vi "FeedbackDecode_SetMvntBuilder.vi"(2 "MvntBuilderIn":T1={"MvntType"={"Thumb"=enum."True", "Index"=enum."False", "Middle"=enum."False", "Ring"=enum."False", "Little"=enum."False", "ThumbInt"=enum."False", "IndexInt"=enum."False", "RingInt"=enum."False", "LittleInt"=enum."False", "WristPitch"=enum."False", "WristYaw"=enum."False", "WristRoll"=enum."False"}, "MvntParams"={"Amp"=1.0, "Delay"=0.0, "Rise"=1.0, "Hold"=1.0}, "MvntList"=[{"MvntMat"=[[1.0, 0.0, 1.0, 1.0], [0.0, 0.0, 0.0, 0.0], [0.0, 0.0, 0.0, 0.0], [0.0, 0.0, 0.0, 0.0], [0.0, 0.0, 0.0, 0.0], [0.0, 0.0, 0.0, 0.0], [0.0, 0.0, 0.0, 0.0], [0.0, 0.0, 0.0, 0.0], [0.0, 0.0, 0.0, 0.0], [0.0, 0.0, 0.0, 0.0], [0.0, 0.0, 0.0, 0.0], [0.0, 0.0, 0.0, 0.0]], "MvntName"="ThumbFlex", "Tracking"=enum."False", "Radius"=0.15}, {"MvntMat"=[[0.0, 0.0, 0.0, 0.0], [1.0, 0.0, 2.0, 2.0], [0.0, 0.0, 0.0, 0.0], [0.0, 0.0, 0.0, 0.0], [0.0, 0.0, 0.0, 0.0], [0.0, 0.0, 0.0, 0.0], [0.0, 0.0, 0.0, 0.0], [0.0, 0.0, 0.0, 0.0], [0.0, 0.0, 0.0, 0.0], [0.0, 0.0, 0.0, 0.0], [0.0, 0.0, 0.0, 0.0], [0.0, 0.0, 0.0, 0.0]], "MvntName"="IndexFlex", "Tracking"=enum."True", "Radius"=0.15}, {"MvntMat"=[[0.0, 0.0, 0.0, 0.0], [0.0, 0.0, 0.0, 0.0], [1.0, 0.0, 1.0, 1.0], [0.0, 0.0, 0.0, 0.0], [0.0, 0.0, 0.0, 0.0], [0.0, 0.0, 0.0, 0.0], [0.0, 0.0, 0.0, 0.0], [0.0, 0.0, 0.0, 0.0], [0.0, 0.0, 0.0, 0.0], [0.0, 0.0, 0.0, 0.0], [0.0, 0.0, 0.0, 0.0], [0.0, 0.0, 0.0, 0.0]], "MvntName"="MiddleFlex", "Tracking"=enum."False", "Radius"=0.15}, {"MvntMat"=[[0.0, 0.0, 0.0, 0.0], [0.0, 0.0, 0.0, 0.0], [0.0, 0.0, 0.0, 0.0], [1.0, 0.0, 1.0, 1.0], [0.0, 0.0, 0.0, 0.0], [0.0, 0.0, 0.0, 0.0], [0.0, 0.0, 0.0, 0.0], [0.0, 0.0, 0.0, 0.0], [0.0, 0.0, 0.0, 0.0], [0.0, 0.0, 0.0, 0.0], [0.0, 0.0, 0.0, 0.0], [0.0, 0.0, 0.0, 0.0]], "MvntName"="RingFlex", "Tracking"=enum."False", "Radius"=0.15}, {"MvntMat"=[[0.0, 0.0, 0.0, 0.0], [0.0, 0.0, 0.0, 0.0], [0.0, 0.0, 0.0, 0.0], [0.0, 0.0, 0.0, 0.0], [1.0, 0.0, 1.0, 1.0], [0.0, 0.0, 0.0, 0.0], [0.0, 0.0, 0.0, 0.0], [0.0, 0.0, 0.0, 0.0], [0.0, 0.0, 0.0, 0.0], [0.0, 0.0, 0.0, 0.0], [0.0, 0.0, 0.0, 0.0], [0.0, 0.0, 0.0, 0.0]], "MvntName"="LittleFlex", "Tracking"=enum."False", "Radius"=0.15}, {"MvntMat"=[[0.0, 0.0, 0.0, 0.0], [0.0, 0.0, 0.0, 0.0], [0.0, 0.0, 0.0, 0.0], [0.0, 0.0, 0.0, 0.0], [0.0, 0.0, 0.0, 0.0], [1.0, 0.0, 1.0, 1.0], [0.0, 0.0, 0.0, 0.0], [0.0, 0.0, 0.0, 0.0], [0.0, 0.0, 0.0, 0.0], [0.0, 0.0, 0.0, 0.0], [0.0, 0.0, 0.0, 0.0], [0.0, 0.0, 0.0, 0.0]], "MvntName"="ThumbInt", "Tracking"=enum."False", "Radius"=0.15}, {"MvntMat"=[[0.0, 0.0, 0.0, 0.0], [0.0, 0.0, 0.0, 0.0], [0.0, 0.0, 0.0, 0.0], [0.0, 0.0, 0.0, 0.0], [0.0, 0.0, 0.0, 0.0], [0.0, 0.0, 0.0, 0.0], [1.0, 0.0, 1.0, 1.0], [0.0, 0.0, 0.0, 0.0], [0.0, 0.0, 0.0, 0.0], [0.0, 0.0, 0.0, 0.0], [0.0, 0.0, 0.0, 0.0], [0.0, 0.0, 0.0, 0.0]], "MvntName"="IndexInt", "Tracking"=enum."False", "Radius"=0.15}, {"MvntMat"=[[0.0, 0.0, 0.0, 0.0], [0.0, 0.0, 0.0, 0.0], [0.0, 0.0, 0.0, 0.0], [0.0, 0.0, 0.0, 0.0], [0.0, 0.0, 0.0, 0.0], [0.0, 0.0, 0.0, 0.0], [0.0, 0.0, 0.0, 0.0], [1.0, 0.0, 1.0, 1.0], [0.0, 0.0, 0.0, 0.0], [0.0, 0.0, 0.0, 0.0], [0.0, 0.0, 0.0, 0.0], [0.0, 0.0, 0.0, 0.0]], "MvntName"="RingInt", "Tracking"=enum."False", "Radius"=0.15}, {"MvntMat"=[[0.0, 0.0, 0.0, 0.0], [0.0, 0.0, 0.0, 0.0], [0.0, 0.0, 0.0, 0.0], [0.0, 0.0, 0.0, 0.0], [0.0, 0.0, 0.0, 0.0], [0.0, 0.0, 0.0, 0.0], [0.0, 0.0, 0.0, 0.0], [0.0, 0.0, 0.0, 0.0], [1.0, 0.0, 1.0, 1.0], [0.0, 0.0, 0.0, 0.0], [0.0, 0.0, 0.0, 0.0], [0.0, 0.0, 0.0, 0.0]], "MvntName"="LittleInt", "Tracking"=enum."False", "Radius"=0.15}, {"MvntMat"=[[0.0, 0.0, 0.0, 0.0], [0.0, 0.0, 0.0, 0.0], [0.0, 0.0, 0.0, 0.0], [0.0, 0.0, 0.0, 0.0], [0.0, 0.0, 0.0, 0.0], [0.0, 0.0, 0.0, 0.0], [0.0, 0.0, 0.0, 0.0], [0.0, 0.0, 0.0, 0.0], [0.0, 0.0, 0.0, 0.0], [1.0, 0.0, 1.0, 1.0], [0.0, 0.0, 0.0, 0.0], [0.0, 0.0, 0.0, 0.0]], "MvntName"="WristPitch", "Tracking"=enum."False", "Radius"=0.15}, {"MvntMat"=[[0.0, 0.0, 0.0, 0.0], [0.0, 0.0, 0.0, 0.0], [0.0, 0.0, 0.0, 0.0], [0.0, 0.0, 0.0, 0.0], [0.0, 0.0, 0.0, 0.0], [0.0, 0.0, 0.0, 0.0], [0.0, 0.0, 0.0, 0.0], [0.0, 0.0, 0.0, 0.0], [0.0, 0.0, 0.0, 0.0], [0.0, 0.0, 0.0, 0.0], [1.0, 0.0, 1.0, 1.0], [0.0, 0.0, 0.0, 0.0]], "MvntName"="WristYaw", "Tracking"=enum."False", "Radius"=0.15}, {"MvntMat"=[[0.0, 0.0, 0.0, 0.0], [0.0, 0.0, 0.0, 0.0], [0.0, 0.0, 0.0, 0.0], [0.0, 0.0, 0.0, 0.0], [0.0, 0.0, 0.0, 0.0], [0.0, 0.0, 0.0, 0.0], [0.0, 0.0, 0.0, 0.0], [0.0, 0.0, 0.0, 0.0], [0.0, 0.0, 0.0, 0.0], [0.0, 0.0, 0.0, 0.0], [0.0, 0.0, 0.0, 0.0], [1.0, 0.0, 1.0, 1.0]], "MvntName"="WristRoll", "Tracking"=enum."False", "Radius"=0.15}], "Set"=FALSE, "Clear"=FALSE, "Load"=FALSE, "Mode"=enum."Selected", "NTrials"=0.0, "TargParams"={"Gain"=1.0, "Radius"=0.15, "Acc"=0.8}, "Save"=FALSE, "PercTrials"=1.0} caption="Movement Builder" {"PercTrials" format="%#_2g"; "NTrials" min=1.0 max=100.0 step=1.0; "MvntList"."Radius" min=0.0 max=1.0 step=0.01; "TargParams"."Acc" min=0.0 max=1.0 step=0.01; "TargParams"."Radius" min=0.0 max=1.0 step=0.01; "TargParams"."Gain" min=-1.0 max=1.0 step=0.01; "MvntParams"."Hold" min=0.0 step=0.1; "MvntParams"."Rise" min=0.0 step=0.1; "MvntParams"."Delay" min=0.0 step=0.1; "MvntParams"."Amp" min=-1.0 max=1.0 step=0.1}, 3 "MvntIdx":i32) -> (0 "MvntBuilderOut":T1={"MvntType"={"Thumb"=enum."True", "Index"=enum."False", "Middle"=enum."False", "Ring"=enum."False", "Little"=enum."False", "ThumbInt"=enum."False", "IndexInt"=enum."False", "RingInt"=enum."False", "LittleInt"=enum."False", "WristPitch"=enum."False", "WristYaw"=enum."False", "WristRoll"=enum."False"}, "MvntParams"={"Amp"=1.0, "Delay"=0.0, "Rise"=1.0, "Hold"=1.0}, "MvntList"=[{"MvntMat"=[[1.0, 0.0, 1.0, 1.0], [0.0, 0.0, 0.0, 0.0], [0.0, 0.0, 0.0, 0.0], [0.0, 0.0, 0.0, 0.0], [0.0, 0.0, 0.0, 0.0], [0.0, 0.0, 0.0, 0.0], [0.0, 0.0, 0.0, 0.0], [0.0, 0.0, 0.0, 0.0], [0.0, 0.0, 0.0, 0.0], [0.0, 0.0, 0.0, 0.0], [0.0, 0.0, 0.0, 0.0], [0.0, 0.0, 0.0, 0.0]], "MvntName"="ThumbFlex", "Tracking"=enum."False", "Radius"=0.15}, {"MvntMat"=[[0.0, 0.0, 0.0, 0.0], [1.0, 0.0, 2.0, 2.0], [0.0, 0.0, 0.0, 0.0], [0.0, 0.0, 0.0, 0.0], [0.0, 0.0, 0.0, 0.0], [0.0, 0.0, 0.0, 0.0], [0.0, 0.0, 0.0, 0.0], [0.0, 0.0, 0.0, 0.0], [0.0, 0.0, 0.0, 0.0], [0.0, 0.0, 0.0, 0.0], [0.0, 0.0, 0.0, 0.0], [0.0, 0.0, 0.0, 0.0]], "MvntName"="IndexFlex", "Tracking"=enum."True", "Radius"=0.15}, {"MvntMat"=[[0.0, 0.0, 0.0, 0.0], [0.0, 0.0, 0.0, 0.0], [1.0, 0.0, 1.0, 1.0], [0.0, 0.0, 0.0, 0.0], [0.0, 0.0, 0.0, 0.0], [0.0, 0.0, 0.0, 0.0], [0.0, 0.0, 0.0, 0.0], [0.0, 0.0, 0.0, 0.0], [0.0, 0.0, 0.0, 0.0], [0.0, 0.0, 0.0, 0.0], [0.0, 0.0, 0.0, 0.0], [0.0, 0.0, 0.0, 0.0]], "MvntName"="MiddleFlex", "Tracking"=enum."False", "Radius"=0.15}, {"MvntMat"=[[0.0, 0.0, 0.0, 0.0], [0.0, 0.0, 0.0, 0.0], [0.0, 0.0, 0.0, 0.0], [1.0, 0.0, 1.0, 1.0], [0.0, 0.0, 0.0, 0.0], [0.0, 0.0, 0.0, 0.0], [0.0, 0.0, 0.0, 0.0], [0.0, 0.0, 0.0, 0.0], [0.0, 0.0, 0.0, 0.0], [0.0, 0.0, 0.0, 0.0], [0.0, 0.0, 0.0, 0.0], [0.0, 0.0, 0.0, 0.0]], "MvntName"="RingFlex", "Tracking"=enum."False", "Radius"=0.15}, {"MvntMat"=[[0.0, 0.0, 0.0, 0.0], [0.0, 0.0, 0.0, 0.0], [0.0, 0.0, 0.0, 0.0], [0.0, 0.0, 0.0, 0.0], [1.0, 0.0, 1.0, 1.0], [0.0, 0.0, 0.0, 0.0], [0.0, 0.0, 0.0, 0.0], [0.0, 0.0, 0.0, 0.0], [0.0, 0.0, 0.0, 0.0], [0.0, 0.0, 0.0, 0.0], [0.0, 0.0, 0.0, 0.0], [0.0, 0.0, 0.0, 0.0]], "MvntName"="LittleFlex", "Tracking"=enum."False", "Radius"=0.15}, {"MvntMat"=[[0.0, 0.0, 0.0, 0.0], [0.0, 0.0, 0.0, 0.0], [0.0, 0.0, 0.0, 0.0], [0.0, 0.0, 0.0, 0.0], [0.0, 0.0, 0.0, 0.0], [1.0, 0.0, 1.0, 1.0], [0.0, 0.0, 0.0, 0.0], [0.0, 0.0, 0.0, 0.0], [0.0, 0.0, 0.0, 0.0], [0.0, 0.0, 0.0, 0.0], [0.0, 0.0, 0.0, 0.0], [0.0, 0.0, 0.0, 0.0]], "MvntName"="ThumbInt", "Tracking"=enum."False", "Radius"=0.15}, {"MvntMat"=[[0.0, 0.0, 0.0, 0.0], [0.0, 0.0, 0.0, 0.0], [0.0, 0.0, 0.0, 0.0], [0.0, 0.0, 0.0, 0.0], [0.0, 0.0, 0.0, 0.0], [0.0, 0.0, 0.0, 0.0], [1.0, 0.0, 1.0, 1.0], [0.0, 0.0, 0.0, 0.0], [0.0, 0.0, 0.0, 0.0], [0.0, 0.0, 0.0, 0.0], [0.0, 0.0, 0.0, 0.0], [0.0, 0.0, 0.0, 0.0]], "MvntName"="IndexInt", "Tracking"=enum."False", "Radius"=0.15}, {"MvntMat"=[[0.0, 0.0, 0.0, 0.0], [0.0, 0.0, 0.0, 0.0], [0.0, 0.0, 0.0, 0.0], [0.0, 0.0, 0.0, 0.0], [0.0, 0.0, 0.0, 0.0], [0.0, 0.0, 0.0, 0.0], [0.0, 0.0, 0.0, 0.0], [1.0, 0.0, 1.0, 1.0], [0.0, 0.0, 0.0, 0.0], [0.0, 0.0, 0.0, 0.0], [0.0, 0.0, 0.0, 0.0], [0.0, 0.0, 0.0, 0.0]], "MvntName"="RingInt", "Tracking"=enum."False", "Radius"=0.15}, {"MvntMat"=[[0.0, 0.0, 0.0, 0.0], [0.0, 0.0, 0.0, 0.0], [0.0, 0.0, 0.0, 0.0], [0.0, 0.0, 0.0, 0.0], [0.0, 0.0, 0.0, 0.0], [0.0, 0.0, 0.0, 0.0], [0.0, 0.0, 0.0, 0.0], [0.0, 0.0, 0.0, 0.0], [1.0, 0.0, 1.0, 1.0], [0.0, 0.0, 0.0, 0.0], [0.0, 0.0, 0.0, 0.0], [0.0, 0.0, 0.0, 0.0]], "MvntName"="LittleInt", "Tracking"=enum."False", "Radius"=0.15}, {"MvntMat"=[[0.0, 0.0, 0.0, 0.0], [0.0, 0.0, 0.0, 0.0], [0.0, 0.0, 0.0, 0.0], [0.0, 0.0, 0.0, 0.0], [0.0, 0.0, 0.0, 0.0], [0.0, 0.0, 0.0, 0.0], [0.0, 0.0, 0.0, 0.0], [0.0, 0.0, 0.0, 0.0], [0.0, 0.0, 0.0, 0.0], [1.0, 0.0, 1.0, 1.0], [0.0, 0.0, 0.0, 0.0], [0.0, 0.0, 0.0, 0.0]], "MvntName"="WristPitch", "Tracking"=enum."False", "Radius"=0.15}, {"MvntMat"=[[0.0, 0.0, 0.0, 0.0], [0.0, 0.0, 0.0, 0.0], [0.0, 0.0, 0.0, 0.0], [0.0, 0.0, 0.0, 0.0], [0.0, 0.0, 0.0, 0.0], [0.0, 0.0, 0.0, 0.0], [0.0, 0.0, 0.0, 0.0], [0.0, 0.0, 0.0, 0.0], [0.0, 0.0, 0.0, 0.0], [0.0, 0.0, 0.0, 0.0], [1.0, 0.0, 1.0, 1.0], [0.0, 0.0, 0.0, 0.0]], "MvntName"="WristYaw", "Tracking"=enum."False", "Radius"=0.15}, {"MvntMat"=[[0.0, 0.0, 0.0, 0.0], [0.0, 0.0, 0.0, 0.0], [0.0, 0.0, 0.0, 0.0], [0.0, 0.0, 0.0, 0.0], [0.0, 0.0, 0.0, 0.0], [0.0, 0.0, 0.0, 0.0], [0.0, 0.0, 0.0, 0.0], [0.0, 0.0, 0.0, 0.0], [0.0, 0.0, 0.0, 0.0], [0.0, 0.0, 0.0, 0.0], [0.0, 0.0, 0.0, 0.0], [1.0, 0.0, 1.0, 1.0]], "MvntName"="WristRoll", "Tracking"=enum."False", "Radius"=0.15}], "Set"=FALSE, "Clear"=FALSE, "Load"=FALSE, "Mode"=enum."Selected", "NTrials"=0.0, "TargParams"={"Gain"=1.0, "Radius"=0.15, "Acc"=0.8}, "Save"=FALSE, "PercTrials"=1.0} caption="Movement Builder" {"PercTrials" format="%#_2g"; "NTrials" min=1.0 max=100.0 step=1.0; "MvntList"."Radius" min=0.0 max=1.0 step=0.01; "TargParams"."Acc" min=0.0 max=1.0 step=0.01; "TargParams"."Radius" min=0.0 max=1.0 step=0.01; "TargParams"."Gain" min=-1.0 max=1.0 step=0.01; "MvntParams"."Hold" min=0.0 step=0.1; "MvntParams"."Rise" min=0.0 step=0.1; "MvntParams"."Delay" min=0.0 step=0.1; "MvntParams"."Amp" min=-1.0 max=1.0 step=0.1})   [LabVIEW 2020]
uses:
  FeedbackDecode_MvntClust.ctl
panel:
  # "Thumb"
  # "Index"
  # "Middle"
  # "Ring"
  # "Little"
  # "ThumbInt"
  # "IndexInt"
  # "RingInt"
  # "LittleInt"
  # "WristPitch"
  # "WristYaw"
  # "WristRoll"
  # "Amp"
  # "Del"
  # "Rise"
  # "Hold"
  # "Thumb"
  # "Index"
  # "Middle"
  # "Ring"
  # "Little"
  # "ThumbInt"
  # "IndexInt"
  # "RingInt"
  # "LittleInt"
  # "WristPitch"
  # "WristYaw"
  # "WristRoll"
  # "Amp"
  # "Del"
  # "Rise"
  # "Hold"
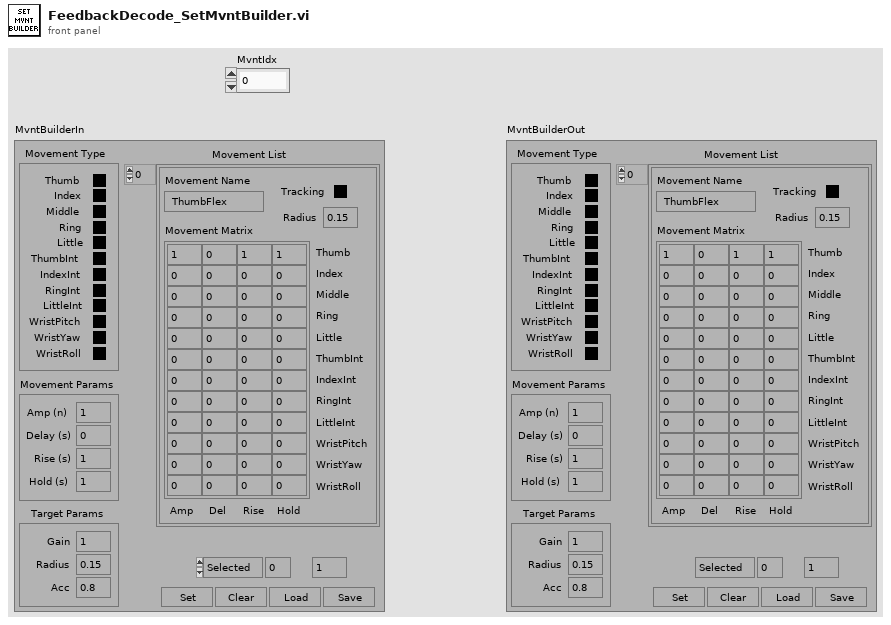
[diagram p1: front panel]
types:
  T1 = typedef "FeedbackDecode_MvntClust.ctl" = cluster{"MvntType":cluster{"Thumb":enum8{"False", "True", "Mixed"}, "Index":enum8{"False", "True", "Mixed"}, "Middle":enum8{"False", "True", "Mixed"}, "Ring":enum8{"False", "True", "Mixed"}, "Little":enum8{"False", "True", "Mixed"}, "ThumbInt":enum8{"False", "True", "Mixed"}, "IndexInt":enum8{"False", "True", "Mixed"}, "RingInt":enum8{"False", "True", "Mixed"}, "LittleInt":enum8{"False", "True", "Mixed"}, "WristPitch":enum8{"False", "True", "Mixed"}, "WristYaw":enum8{"False", "True", "Mixed"}, "WristRoll":enum8{"False", "True", "Mixed"}}, "MvntParams":cluster{"Amp":dbl, "Delay":dbl, "Rise":dbl, "Hold":dbl}, "MvntList":cluster{"MvntMat":dbl[][], "MvntName":string, "Tracking":enum8{"False", "True", "Mixed"}, "Radius":dbl}[], "Set":bool, "Clear":bool, "Load":bool, "Mode":enum16{"Selected", "Block", "Random"}, "NTrials":dbl, "TargParams":cluster{"Gain":dbl, "Radius":dbl, "Acc":dbl}, "Save":bool, "PercTrials":dbl}
  T2 = cluster{"Thumb":enum8{"False", "True", "Mixed"}, "Index":enum8{"False", "True", "Mixed"}, "Middle":enum8{"False", "True", "Mixed"}, "Ring":enum8{"False", "True", "Mixed"}, "Little":enum8{"False", "True", "Mixed"}, "ThumbInt":enum8{"False", "True", "Mixed"}, "IndexInt":enum8{"False", "True", "Mixed"}, "RingInt":enum8{"False", "True", "Mixed"}, "LittleInt":enum8{"False", "True", "Mixed"}, "WristPitch":enum8{"False", "True", "Mixed"}, "WristYaw":enum8{"False", "True", "Mixed"}, "WristRoll":enum8{"False", "True", "Mixed"}}
  T3 = cluster{"Amp":dbl, "Delay":dbl, "Rise":dbl, "Hold":dbl}
  T4 = cluster{"MvntMat":dbl[][], "MvntName":string, "Tracking":enum8{"False", "True", "Mixed"}, "Radius":dbl}[]
  T5 = cluster{"MvntMat":dbl[][], "MvntName":string, "Tracking":enum8{"False", "True", "Mixed"}, "Radius":dbl}
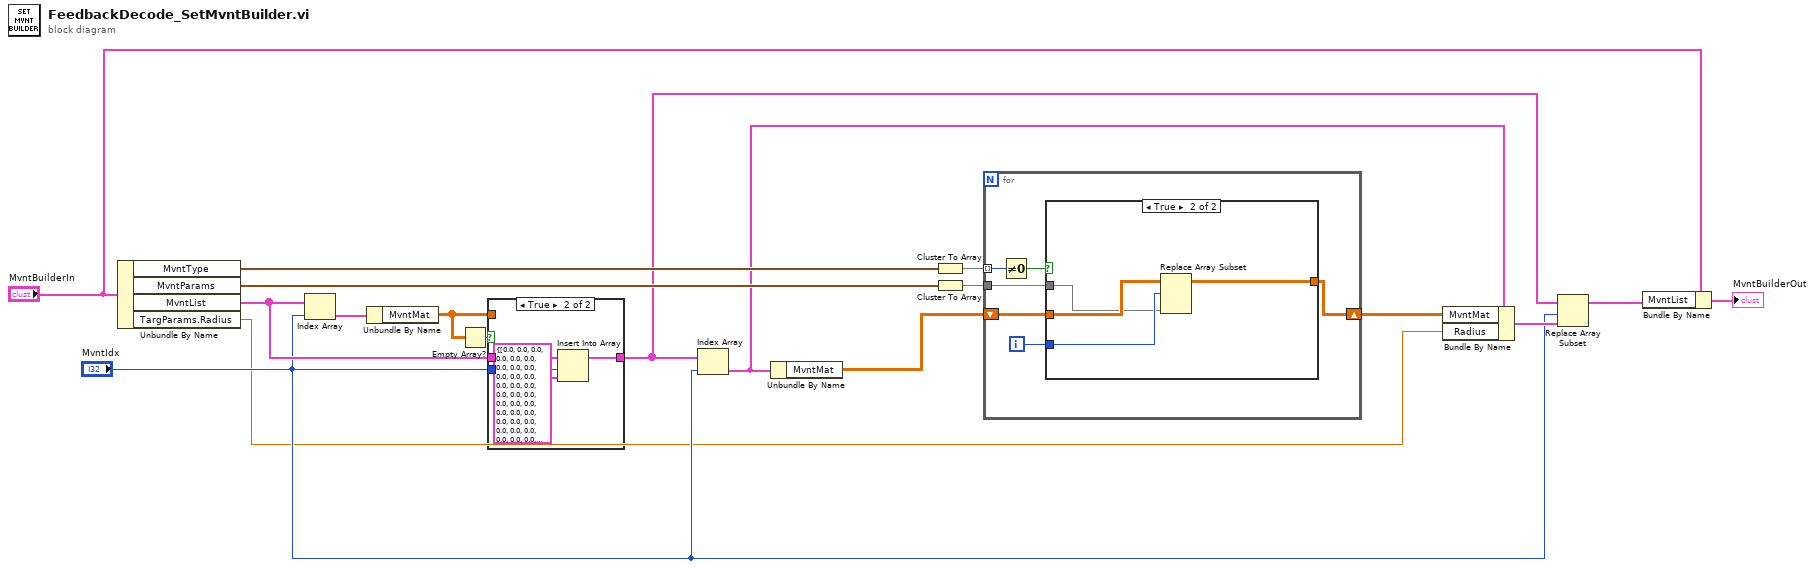
[diagram p0: block diagram]
diagram:
  n1 = Unbundle By Name("MvntBuilderIn") -> ("MvntType"=w18:T2, "MvntParams"=w16:T3, "MvntList"=w8:T4, "TargParams.Radius"=w1:dbl)
  n2 = Index Array(array=w8, index="MvntIdx") -> (element=w14:T5)
  n3 = Unbundle By Name(w14) -> ("MvntMat"=w9:dbl[][])
  n4 = Empty Array?(array=w9) -> (empty?=w10:bool)
  n5 = case shown="True" w10 {
    tunnel: w9 -> [_ _]
    tunnel: w8 -> [w19 w23]
    tunnel: "MvntIdx" -> [_ w22]
    tunnel: [w19 w21] -> w7
    frame False {
    }
    frame True {
      n6 = Insert Into Array(array=w23, index=w22, new element=T5 {"MvntMat"=[[0.0, 0.0, 0.0, 0.0], [0.0, 0.0, 0.0, 0.0], [0.0, 0.0, 0.0, 0.0], [0.0, 0.0, 0.0, 0.0], [0.0, 0.0, 0.0, 0.0], [0.0, 0.0, 0.0, 0.0], [0.0, 0.0, 0.0, 0.0], [0.0, 0.0, 0.0, 0.0], [0.0, 0.0, 0.0, 0.0], [0.0, 0.0, 0.0, 0.0], [0.0, 0.0, 0.0, 0.0], [0.0, 0.0, 0.0, 0.0]], "MvntName"="", "Tracking"=enum."False", "Radius"=0.15} ("new element/subarray")) -> (w21:T4)
    }
  }
  n7 = Index Array(array=w7, index="MvntIdx") -> (element=w5:T5)
  n8 = Unbundle By Name(w5) -> ("MvntMat"=w6:dbl[][])
  n9 = Cluster To Array(cluster=w18) -> (array=w17:enum8{"False", "True", "Mixed"}[])
  n10 = Cluster To Array(cluster=w16) -> (array=w15:dbl[])
  n11 = for {
    tunnel: w17 -> [w29] mode=indexing
    shift-right: [w24] -> w13
    shift-left: w6 -> [w27]
    tunnel: w15 -> [w25]
    i -> [w26]
    n12 = Not Equal To 0?(x=w29) -> (x != 0?=w28:bool)
    n13 = case shown="True" w28 {
      tunnel: w27 -> [w30 w34]
      tunnel: w26 -> [_ w33]
      tunnel: w25 -> [_ w32]
      tunnel: [w30 w31] -> w24
      frame False {
      }
      frame True {
        n14 = Replace Array Subset(array=w34, new element=w32, index (row)=w33) -> (w31:dbl[][])  [unwired: 1 in]
      }
    }
  }
  n15 = Bundle By Name(cluster=w5, "MvntMat"=w13, "Radius"=w1) -> (w12:T5)
  n16 = Replace Array Subset(array=w7, new element=w12, index="MvntIdx") -> (w11:T4)
  n17 = Bundle By Name(cluster="MvntBuilderIn", "MvntList"=w11) -> (→"MvntBuilderOut":T1)
